vi "SetTitleBar.vi"(8 "error in (no error)":errorcluster, 11 "WindowFrame in":refnum<class "WindowFrame.lvclass">=refnum) -> (0 "error out":errorcluster, 3 "WindowFrame out":refnum<class "WindowFrame.lvclass">)   [LabVIEW 2020]
uses:
  WindowFrame.lvclass
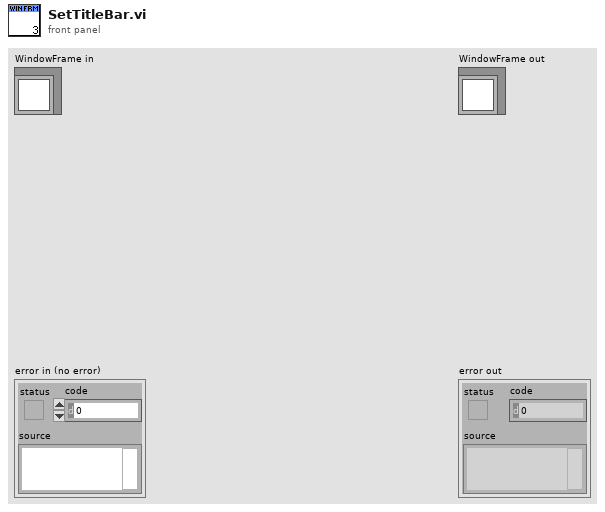
[diagram p1: front panel]
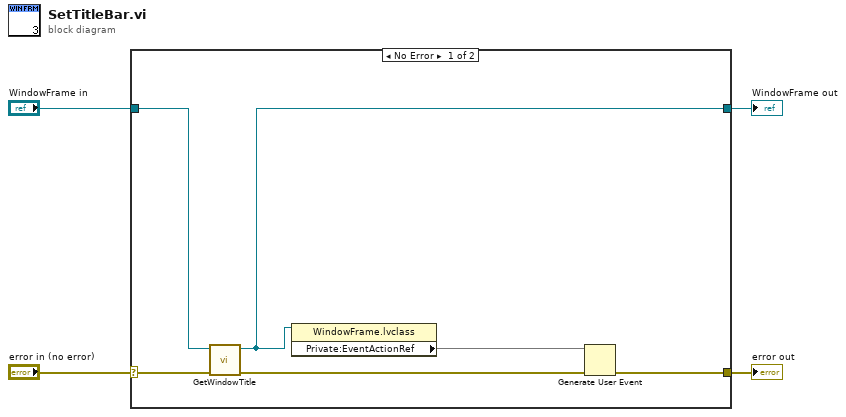
[diagram p0: block diagram]
diagram:
  n1 = case shown="No Error" "error in (no error)" {
    selector: "error in (no error)" -> [w10 w12]
    tunnel: [w5 w12] -> w3
    tunnel: [w8 w11] -> w1
    tunnel: "WindowFrame in" -> [w9 w11]
    frame No Error {
      n2 = call "GetWindowTitle.vi"("error in (no error)"=w10, "WindowFrame in"=w9) -> ("error out"=w6:errorcluster, "WindowFrame out"=w8:refnum<class "WindowFrame.lvclass">)  [unwired: 7 in, 1 out]
      n3 = property class="WindowFrame.lvclass"(reference=w8) -> ("Private:EventActionRef"=w7)  [unwired: 1 in, 2 out]
      n4 = Generate User Event(user event=w7, error in=w6) -> (error out=w5:errorcluster)  [unwired: 2 in, 1 out]
    }
    frame Error {
    }
  }
  "error out" <- w3
  "WindowFrame out" <- w1
